vi "Exercise3.vi"() -> ()   [LabVIEW 2019]
panel:
  out "?":bool
  in  "Turn Off:":timestamp
  in  "Turn On:":timestamp
  out "Current Time":string
  out "Current Date":string
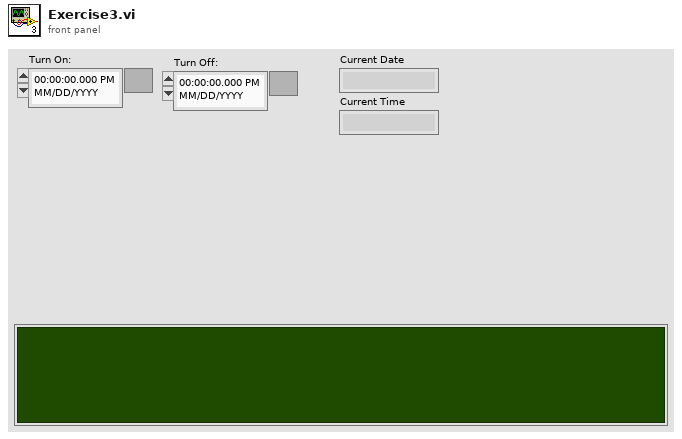
[diagram p1: front panel]
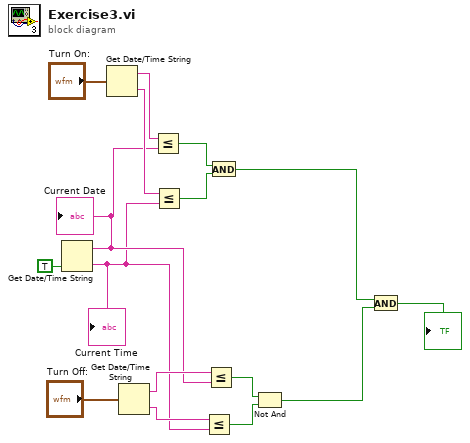
[diagram p0: block diagram]
diagram:
  n1 = Get Date/Time String(want seconds? (F)=TRUE) -> (date string=w7:string, time string=w5:string)  [unwired: 2 in]
  "Current Date" <- w7
  "Current Time" <- w5
  n2 = Get Date/Time String(seconds (now)="Turn On:") -> (date string=w13:string, time string=w12:string)  [unwired: 2 in]
  n3 = Get Date/Time String(seconds (now)="Turn Off:") -> (date string=w8:string, time string=w6:string)  [unwired: 2 in]
  n4 = Less Or Equal?(x=w13, y=w7) -> (x <= y?=w11:bool)
  n5 = Less Or Equal?(x=w12, y=w5) -> (x <= y?=w10:bool)
  n6 = Less Or Equal?(x=w6, y=w5) -> (x <= y?=w2:bool)
  n7 = Less Or Equal?(x=w8, y=w7) -> (x <= y?=w3:bool)
  n8 = And(x=w11, y=w10) -> (x .and. y?=w9:bool)
  n9 = Not And(1:w2, 2:w3) -> (0:w1:bool)
  n10 = And(x=w9, y=w1) -> (x .and. y?=→"?":bool)
